vi "Read Value.vi"(8 "Error In":errorcluster, 11 "String In":refnum<class "String.lvclass">) -> (0 "Error Out":errorcluster, 2 "Value":string, 3 "String Out":refnum<class "String.lvclass">)   [LabVIEW 2018, in "Toolkit.lvlib" / "Data.lvlib" / "String.lvclass"]
uses:
  String.lvclass
  String.lvclass/String.ctl
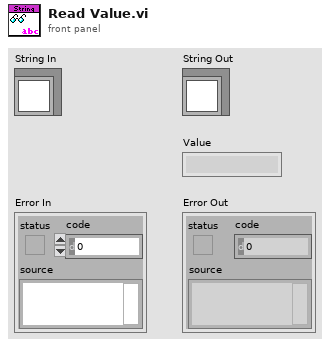
[diagram p1: front panel]
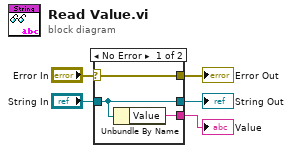
[diagram p0: block diagram]
diagram:
  n1 = case shown="No Error" "Error In" {
    selector: "Error In" -> [w8 w9]
    tunnel: [w8 w9] -> w4
    tunnel: [w7 w10] -> w2
    tunnel: "String In" -> [w7 w10]
    tunnel: [w6 _] -> w1
    frame No Error {
      n2 = Unbundle By Name(w7) -> ("Value"=w6:string)
    }
    frame Error {
    }
  }
  "Error Out" <- w4
  "String Out" <- w2
  "Value" <- w1
